vi "Read TestApplication.vi"(8 "error in (no error)":errorcluster, 11 "TestApplicationError in":refnum<class "TestApplicationError.lvclass">) -> (0 "error out":errorcluster, 2 "TestApplication":refnum<class "TestApplication.lvclass">, 3 "TestApplicationError out":refnum<class "TestApplicationError.lvclass">)   [LabVIEW 2022 SP3, in "Demo.lvlib" / "TestApplicationError.lvclass"]
uses:
  TestApplicationError.lvclass
  TestApplication/TestApplication.lvclass
  TestApplicationError.lvclass/TestApplicationError.ctl
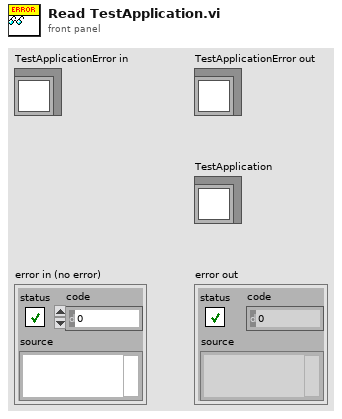
[diagram p1: front panel]
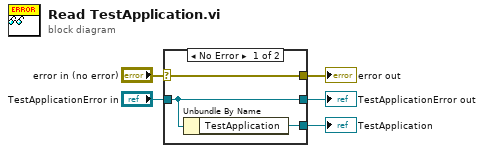
[diagram p0: block diagram]
diagram:
  n1 = case shown="No Error" "error in (no error)" {
    selector: "error in (no error)" -> [w8 w9]
    tunnel: [w8 w9] -> w4
    tunnel: [w7 w10] -> w2
    tunnel: "TestApplicationError in" -> [w7 w10]
    tunnel: [w6 _] -> w1
    frame No Error {
      n2 = Unbundle By Name(w7) -> ("TestApplication"=w6:refnum<class "TestApplication.lvclass">)
    }
    frame Error {
    }
  }
  "error out" <- w4
  "TestApplicationError out" <- w2
  "TestApplication" <- w1
